vi "MagX Get Info.vi"(7 "url":string="http://magx.lanl.gov/rest/now/", 8 "error in":errorcluster, 11 "location":string="Cell_3") -> (0 "error out":errorcluster, 3 "Data out":T1[](array[typedef]))   [LabVIEW 2020]
uses:
  Experiment info.ctl
  7bf855a0-2889-4335-a077-b20b33b30227.vi
  <vilib>/JDP Science/JSONtext/JSON text to Variant.vi
  <vilib>/JDP Science/JSONtext/LVClass Serializer/JSONtext LVClass Serializer.lvclass
  <vilib>/httpClient/LabVIEWHTTPClient.lvlib
panel:
  in  "Experiment info file":path=path "C:/Data/experiment_info.txt"
  in  "Update experiment info file":bool
  in  "Location file":path=path "C:/Data/location.txt"
  out "body":string
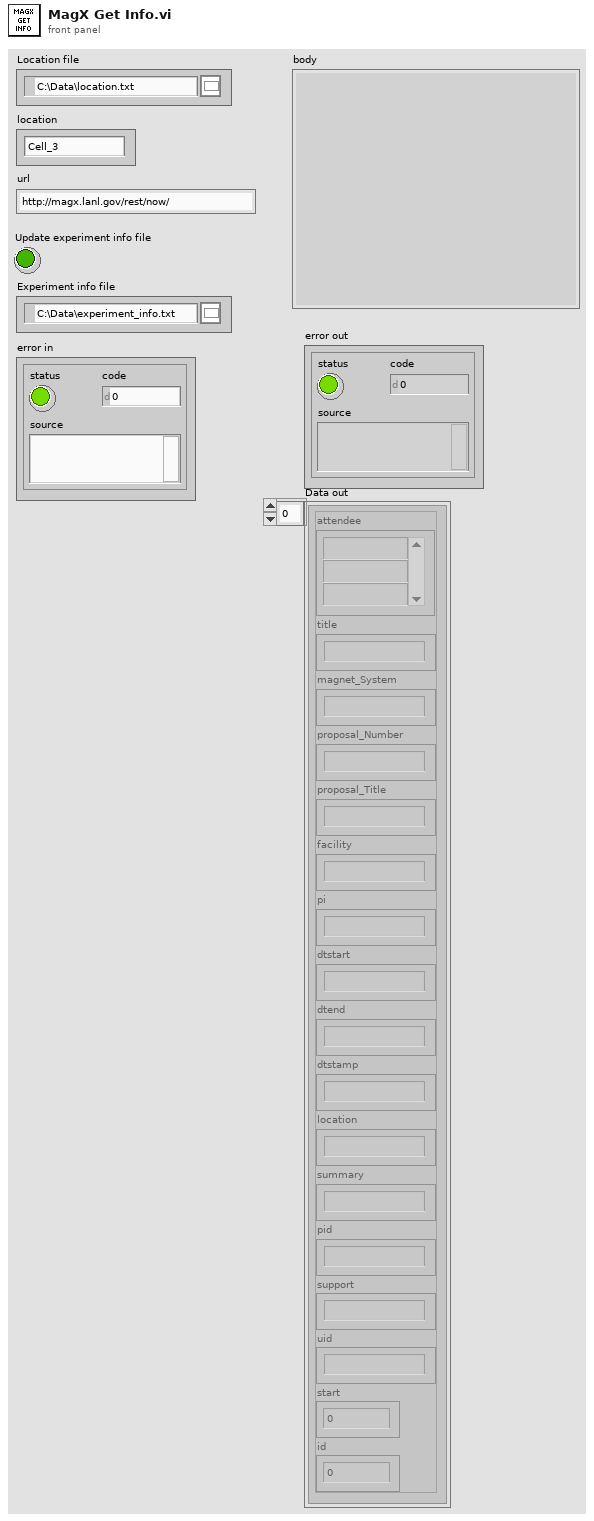
[diagram p1: front panel]
types:
  T1 = typedef "Experiment info.ctl" = cluster{"attendee":string[], "title":string, "magnet_System":string, "proposal_Number":string, "proposal_Title":string, "facility":string, "pi":string, "dtstart":string, "dtend":string, "dtstamp":string, "location":string, "summary":string, "pid":string, "support":string, "uid":string, "start":u64, "id":u64}
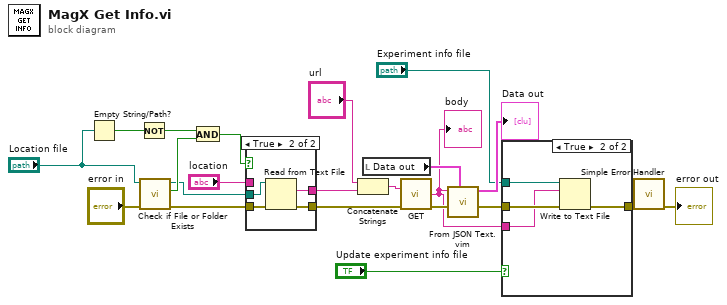
[diagram p0: block diagram]
diagram:
  n1 = Empty String/Path?(string/path="Location file") -> (empty?=w15:bool)
  n2 = Not(x=w15) -> (.not. x?=w14:bool)
  n3 = call <vilib>:"Check if File or Folder Exists.vi"("error in (no error)"="error in", "path"="Location file") -> ("error out"=w9:errorcluster, "file or folder exists?"=w13:bool, "dup path"=w10:path)  [unwired: 7 in]
  n4 = And(x=w14, y=w13) -> (x .and. y?=w12:bool)
  n5 = case shown="True" w12 {
    tunnel: w10 -> [_ w28]
    tunnel: w9 -> [w24 w27]
    tunnel: [w24 w26] -> w7
    tunnel: [w23 w25] -> w8
    tunnel: "location" -> [w23 _]
    frame False {
    }
    frame True {
      n6 = Read from Text File(file (use dialog)=w28, error in=w27) -> (text=w25:string, error out=w26:errorcluster)  [unwired: 2 in, 2 out]
    }
  }
  n7 = Concatenate Strings("url", w8) -> (w18:string)
  n8 = local read "Data out"() -> (w17:T1[])
  n9 = call <vilib>:"GET.vi"("url"=w18, "error in (no error)"=w7) -> ("body"=w1:string, "error out"=w21:errorcluster)  [unwired: 10 in, 2 out]
  "body" <- w1
  n10 = call "From JSON Text.vim"("Data Type and Default Value"=w17, "error in (no error)"=w21, "JSON"=w1) -> ("error out"=w4:errorcluster, "Data out"=→"Data out":T1[])  [unwired: 7 in]
  n11 = case shown="True" "Update experiment info file" {
    tunnel: w4 -> [w29 w33]
    tunnel: "Experiment info file" -> [_ w32]
    tunnel: [w29 w31] -> w2
    tunnel: w1 -> [_ w30]
    frame False {
    }
    frame True {
      n12 = Write to Text File(file (use dialog)=w32, text=w30, error in=w33) -> (error out=w31:errorcluster)  [unwired: 1 in, 2 out]
    }
  }
  n13 = call <vilib>:"Simple Error Handler.vi"("error in (no error)"=w2) -> ("error out"=→"error out":errorcluster)  [unwired: 4 in, 4 out]
